vi "Write ce.vi"(8 "error in (no error)":errorcluster, 10 "ce":dbl[unit] min=-0.00048481368110953597 max=0.00048481368110953597, 11 "CollOffset in":refnum<class "CollOffset.lvclass">) -> (0 "error out":errorcluster, 3 "CollOffset out":refnum<class "CollOffset.lvclass">)   [LabVIEW 2014, in "TCSDataDefinitions.lvlib" / "TCSCommand.lvlib" / "OffsetCommands.lvlib" / "CollOffset.lvclass"]
uses:
  CollOffset.lvclass
  CollOffset.lvclass/CollOffset.ctl
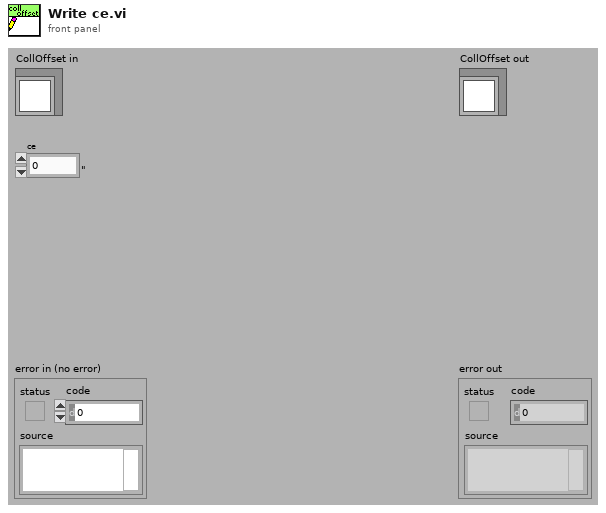
[diagram p1: front panel]
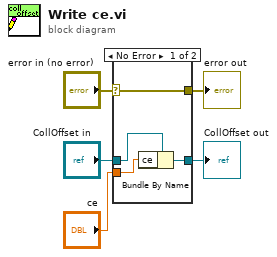
[diagram p0: block diagram]
diagram:
  n1 = case shown="No Error" "error in (no error)" {
    selector: "error in (no error)" -> [w9 w10]
    tunnel: [w9 w10] -> w4
    tunnel: [w7 w11] -> w2
    tunnel: "CollOffset in" -> [w8 w11]
    tunnel: "ce" -> [w6 _]
    frame No Error {
      n2 = Bundle By Name(cluster=w8, "ce"=w6) -> (w7:refnum<class "CollOffset.lvclass">)
    }
    frame Error {
    }
  }
  "error out" <- w4
  "CollOffset out" <- w2
